vi "Demultiplexer_Laser160.vi"() -> ()   [LabVIEW 2012]
uses:
  <vilib>/Platform/TimedLoop/XDataNode/timing_clust.ctl
  <vilib>/Platform/TimedLoop/XDataNode/nitl_modes.ctl
  <vilib>/Platform/TimedLoop/XDataNode/wakeup.ctl
  <vilib>/rvi/Emulation/niFpgaSctlEmulationRegisterWithScheduler.vi
  <vilib>/rvi/eio/common/nirviEmuTemplateMethod_errors.vi
  <vilib>/rvi/Emulation/niFpgaSctlEmulationScheduler.vi
  <vilib>/rvi/FIFO/Fifo_Resource/nirvififoEmulationSetSize.vi
  <vilib>/rvi/DataTransferAndStorage/Container/Common/niFpgaContainerGetUniqueNameForEmu.vi
  <vilib>/rvi/errors/niFpgaSetErrorForExecOnDevCompSimple.vi
  <vilib>/rvi/eio/common/nirviEmuReportErrorAndStop.vi
  <vilib>/rvi/Emulation/niFpgaSctlEmulationFifoFullMgr.vi
  <vilib>/rvi/Emulation/niFpgaSctlEmulationResourceMgr.vi
  <vilib>/rvi/interface/RandomDataEmulation/nirviRandomDataFPGAFIFO.vi
  <vilib>/rvi/interface/RandomDataEmulation/niFpgaRandomDataHandleErrors.vi
  <vilib>/rvi/Emulation/niFpgaSctlEmulationGlobalWrite.vi
  <vilib>/Platform/TimedLoop/XDataNode/XDataNode.xnode
  <vilib>/eio/EIONode/EIONode.xnode
  <vilib>/rvi/DataTransferAndStorage/Container/XNode/niFpgaContainer.xnode
  <vilib>/rvi/FIFO/Fifo_Resource/nirvififoEmulationClear.vi
  <vilib>/rvi/FIFO/Fifo_Resource/nirvififoEmulationWrite.vi
  <vilib>/rvi/FIFO/Fifo_Resource/nirvififoEmulationRead.vi
  <vilib>/rvi/interface/RandomDataEmulation/nirviRandomDataFpgaReadWriteTemplate.vi
  <vilib>/Platform/TimedLoop/XDataNode/XDNodeRunTimeDep.lvlib
panel:
  out "Laser pulse count A1":u16
  out "ToHost FIFO Overflow A2Ch2":bool
  out "ToHost FIFO Overflow A2Ch1":bool
  out "ToHost FIFO Overflow A1Ch2":bool
  in  "Samples per pixel Acq A2":u16=10000 caption="Samples per pixel Acq"
  in  "Samples per pixel Acq A1":u16=10000 caption="Samples per pixel Acq"
  in  "Requested pixels A2":u32=100000 caption="Requested pixels"
  in  "Samples per pixel A2":u16=10000 caption="Samples per pixel"
  out "ToHost FIFO Overflow A1Ch1":bool
  out "Acquiring":bool
  in  "Wait for trigger":bool
  in  "Acquire continuously":bool=TRUE
  in  "Requested pixels A1":u32=100000 caption="Requested pixels"
  in  "Clear Interloop FIFO":bool
  out "Interloop FIFO overflow":bool
  in  "Samples per pixel A1":u16=10000 caption="Samples per pixel"
  in  "Acquire":bool
  out "Interloop FIFO timeout":bool
  in  "Commit":bool
  out "Xpoint_Switch_Ready":bool
  in  "Xpoint_Switch_Write":bool
  in  "Clock Source":u8(ring)=3 items=["Tristate"=0, "Sync Clock (PXIe only)"=2, "Adapter Module Onboard Clock"=3, "Strobe from Crosspoint Switch"=4, "Strobe Bypass"=5]
  in  "Onboard_Clock_Write":bool
  in  "Onboard_Clock_Write_Data":u16
  out "Onboard_Clock_Ready":bool
  in  "Acq_Reset":bool
  # "6587 IO module configuration"
  # "Demultiplexer - Laser 160MHz"
  # "Acquisition control"
  # "Area 1"
  # "Area 2"
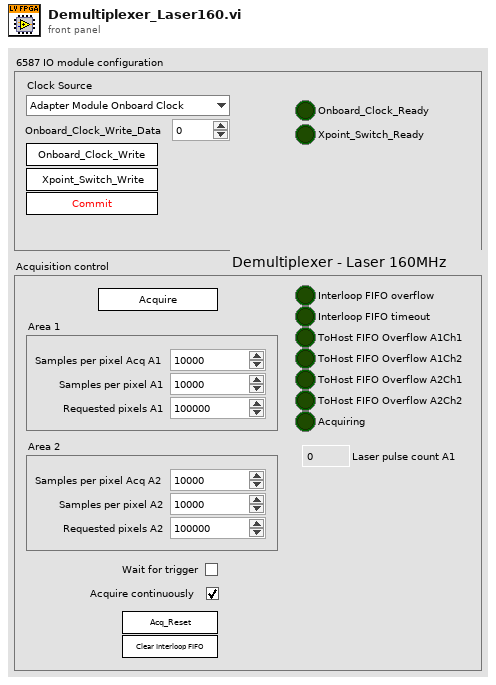
[diagram p1: front panel]
types:
  T1 = typedef "XDNodeRunTimeDep.lvlib/timing_clust.ctl" = cluster{"Expected End [f-1]":u64, "Actual End [f-1]":u64, "Finished Late? [f-1]":bool, "Expected End [i-1]":u64, "Actual End [i-1]":u64, "Finished Late? [i-1]":bool, "Expected Start [i]":u64, "Actual Start [i]":u64, "Expected Start [f]":u64, "Actual Start [f]":u64, "Source Name":string, "Structure Name":string, "Period":i64, "Deadline":i64, "Offset":i64, "Start":i64, "Priority":i32, "Timeout":i32, "Mode":T2, "Wakeup Reason":T3, "Error":errorcluster, "Source Type":string, "Secondary Source Type":string, "Global End Time":u64, "Global Start Time":u64, "Frame Duration":u64, "Iteration Duration":u64, "Assigned CPU":i32, "I/O Scan Engine Mode":u32}
  T2 = typedef "XDNodeRunTimeDep.lvlib/nitl_modes.ctl" = enum32{"No Change", "Process missed periods, maintain original phase", "Discard missed periods, maintain original phase", "Process missed periods, ignore original phase", "Discard missed periods, ignore original phase"}
  T3 = typedef "XDNodeRunTimeDep.lvlib/wakeup.ctl" = enum32{"Normal", "Aborted", "Asynchronous wakeup", "Timing source error", "Timed loop error", "Timeout"}
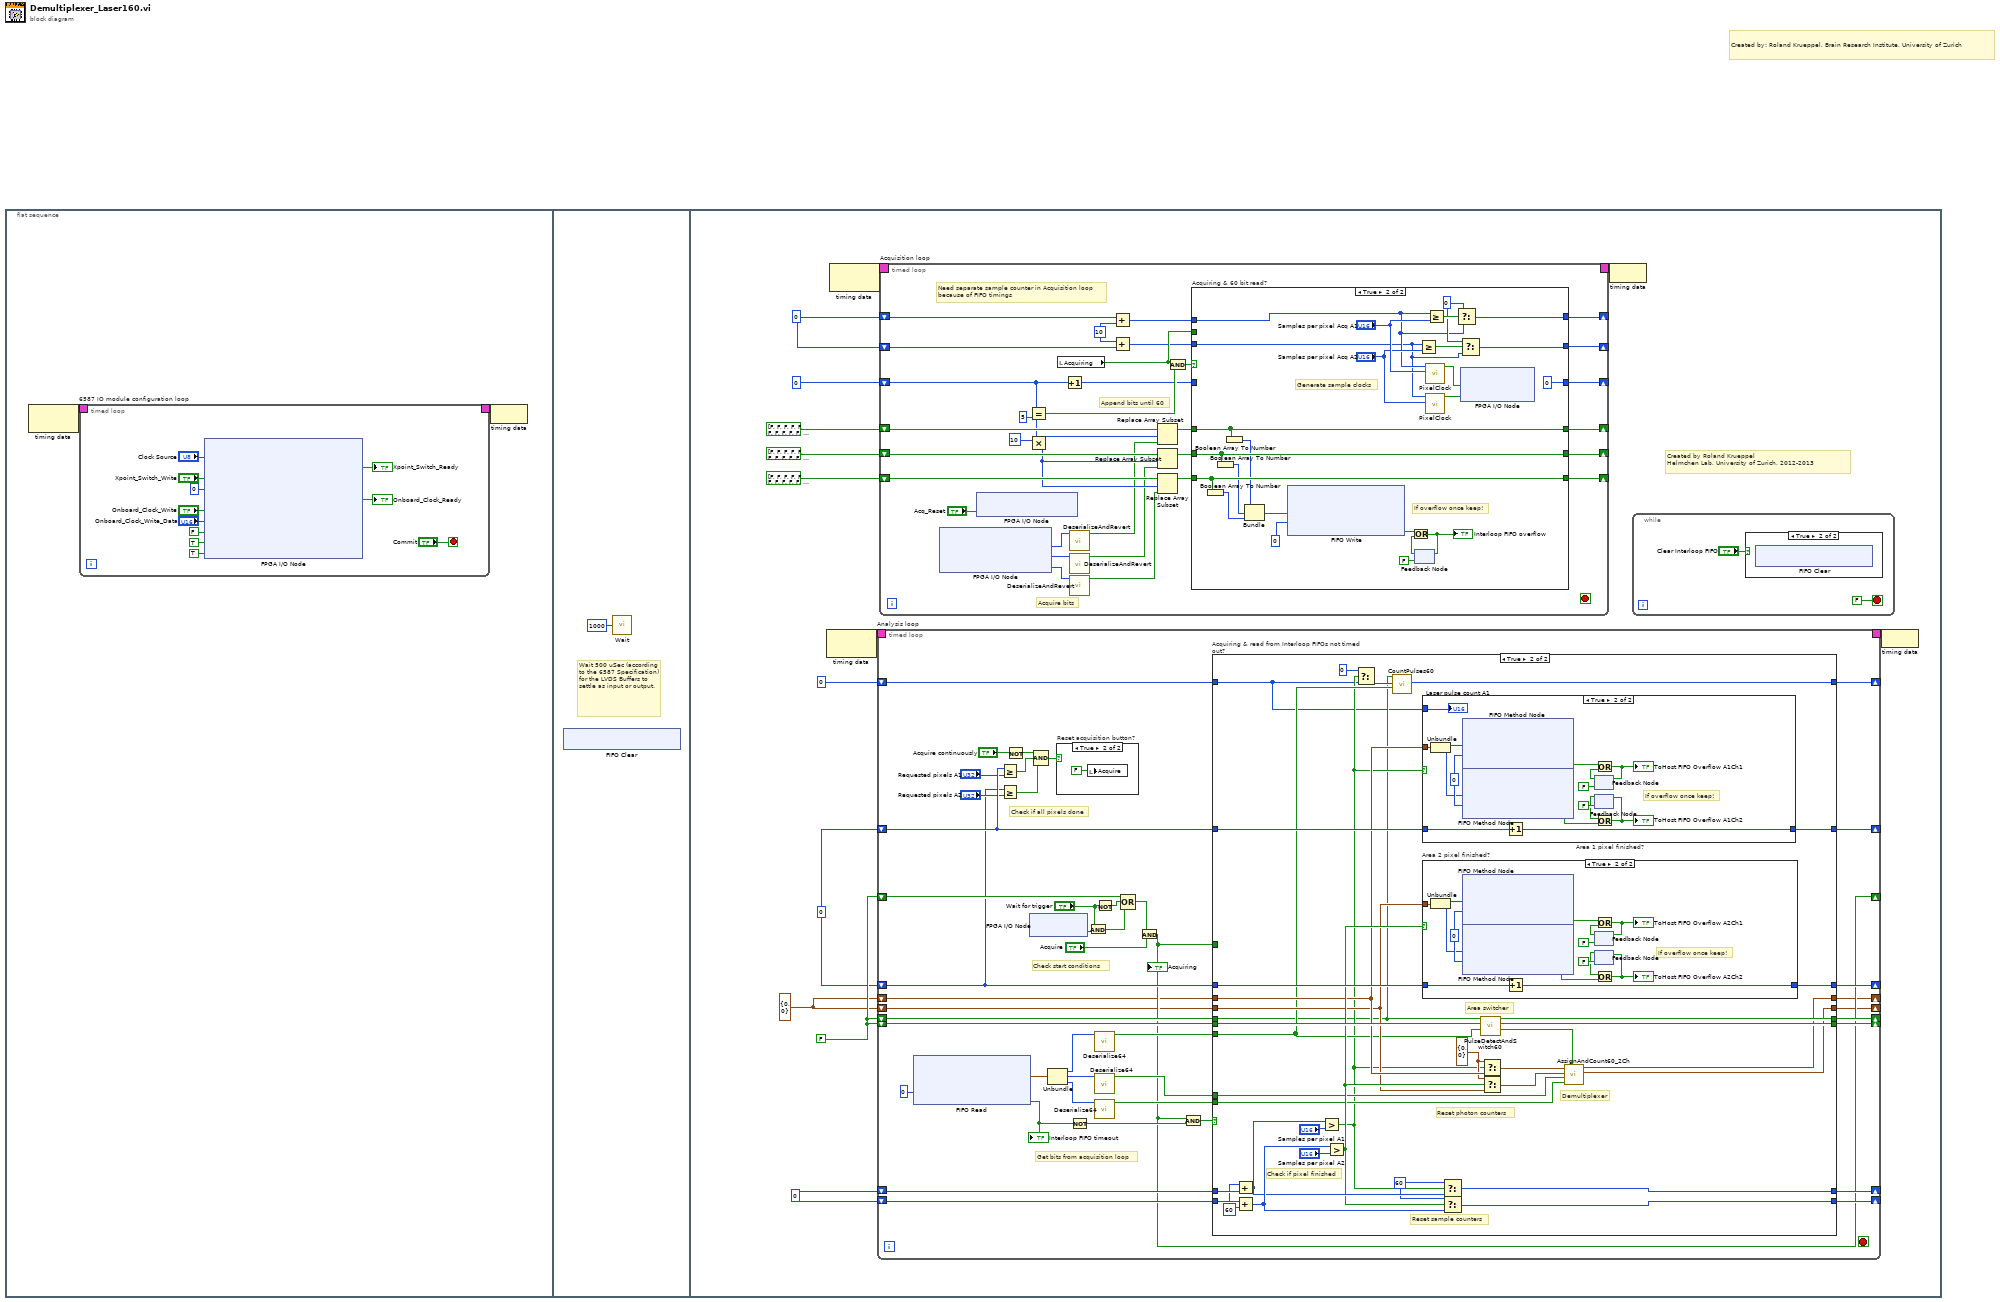
[diagram p0: block diagram]
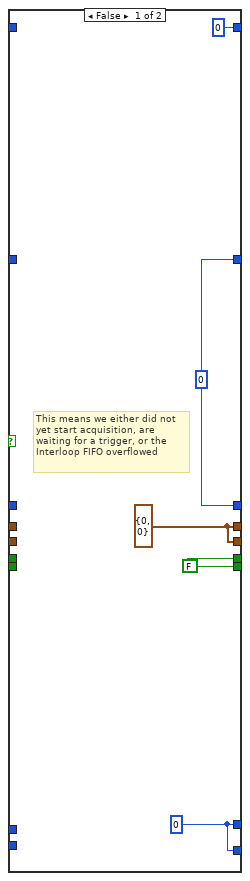
[diagram p5: hidden frame]
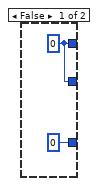
[diagram p9: hidden frame]
diagram:
  # "Created by: Roland Krueppel, Brain Research Institute, University of Zurich"
  n1 = flat-sequence {
    frame #0 {
      n2 = node-c288() -> (w2:T1)  [unwired: 1 in]
      n3 = timed-loop "6587 IO module configuration loop" {
        timing: w2 -> [_]
        timing-out: [_] -> w1
        stop <- "Commit" stop-if-true
        n4 = xnode "FPGA I/O Node"("IO Module\\Acq_IO_Clock_Source"="Clock Source", "IO Module\\Xpoint_Switch_Write"="Xpoint_Switch_Write", "IO Module\\LVDS_Data_Dir"=u16 0 ("IO Module\\LVDS_Data_Dir"), "IO Module\\Onboard_Clock_Write"="Onboard_Clock_Write", "IO Module\\Onboard_Clock_Write_Data"="Onboard_Clock_Write_Data", "IO Module\\SE_PFI0_WE"=FALSE ("IO Module\\SE_PFI0_WE"), "IO Module\\SE_PFI1_WE"=TRUE ("IO Module\\SE_PFI1_WE"), "IO Module\\SE_PFI2_WE"=TRUE ("IO Module\\SE_PFI2_WE")) -> ("IO Module\\Xpoint_Switch_Ready"=→"Xpoint_Switch_Ready":bool, "IO Module\\Onboard_Clock_Ready"=→"Onboard_Clock_Ready":bool)  [unwired: 10 in, 10 out]
      }
      n5 = node-c288(w1) -> ()
    }
    frame #1 {
      # "Wait 500 uSec (according to the 6587 Specification) for the LVDS Buffers to settle as input or output."
      n6 = xnode "FIFO Clear"() -> ()  [unwired: 1 in, 1 out]
      n7 = call "Wait"("Count(uSec)"=u32 1000) -> ()  [unwired: 1 out]
    }
    frame #2 {
      w21 = cluster{u16, u16} {0, 0} ("output cluster")
      w22 = u16 0
      w20 = u32 0 ("Cycle counter out")
      w23 = u16 0
      w24 = FALSE ("Last laser bit out")
      # "Created by Roland Krueppel\nHelmchen Lab, University of Zurich, 2012-2013"
      n8 = node-c288() -> (w30:T1)  [unwired: 1 in]
      n9 = node-c288() -> (w32:T1)  [unwired: 1 in]
      n10 = timed-loop "Analysis loop" {
        timing: w30 -> [_]
        timing-out: [_] -> w29
        shift-right: [w75] -> _
        shift-left: w24 -> [w78]
        shift-right: [w77] -> _
        shift-left: w24 -> [w76]
        shift-right: [w51] -> _
        shift-left: w23 -> [w74]
        shift-right: [w49] -> _
        shift-left: w20 -> [w73]
        shift-right: [w47] -> _
        shift-left: w24 -> [w62]
        shift-right: [w50] -> _
        shift-left: w23 -> [w57]
        shift-right: [w48] -> _
        shift-left: w20 -> [w55]
        shift-right: [w38] -> _
        shift-left: w21 -> [w40]
        shift-right: [w37] -> _
        shift-left: w21 -> [w39]
        shift-right: [w36] -> _
        shift-left: u16 0 ("New pulse count") -> [w35]
        stop <- _ stop-if-true
        # "Get bits from acquisition loop"
        # "Check start conditions"
        # "Check if all pixels done"
        n11 = xnode ("FIFO Read")("Timeout"=0) -> ("Element"=w44:cluster{"Laser":u64, "Ch0":u64, "Ch1":u64}, "Timed Out?"=w45:bool)  [unwired: 1 in, 1 out]
        "Interloop FIFO timeout" <- w45
        n12 = Greater Or Equal?(x=w73, y="Requested pixels A1") -> (x >= y?=w53:bool)
        n13 = Greater Or Equal?(x=w55, y="Requested pixels A2") -> (x >= y?=w52:bool)
        n14 = Not(x="Acquire continuously") -> (.not. x?=w54:bool)
        n15 = xnode "FPGA I/O Node"() -> ("TriggerIn"=w68:bool)  [unwired: 1 in, 1 out]
        n16 = Compound Arithmetic op=AND(w54, w53, w52) -> (w70:bool)
        n17 = Unbundle(w44) -> ("Laser"=w43:u64, "Ch0"=w42:u64, "Ch1"=w41:u64)
        n18 = case "Reset acquisition button?" shown="True" w70 {
          frame False {
          }
          frame True {
            n19 = local write "Acquire"(FALSE ("Acquire")) -> ()
          }
        }
        n20 = Not(x=w45) -> (.not. x?=w63:bool)
        n21 = And(x="Wait for trigger", y=w68) -> (x .and. y?=w65:bool)
        n22 = call "Deserialize64.vi"("U64 input"=w43) -> ("60bit output"=w60:bool[])  [unwired: 10 in]
        n23 = call "Deserialize64.vi"("U64 input"=w42) -> ("60bit output"=w59:bool[])  [unwired: 10 in]
        n24 = call "Deserialize64.vi"("U64 input"=w41) -> ("60bit output"=w58:bool[])  [unwired: 10 in]
        n25 = Not(x="Wait for trigger") -> (.not. x?=w66:bool)
        n26 = Compound Arithmetic op=OR(w62, w66, w65) -> (w64:bool)
        n27 = And(x=w64, y="Acquire") -> (x .and. y?=w47:bool)
        "Acquiring" <- w47
        n28 = And(x=w47, y=w63) -> (x .and. y?=w61:bool)
        n29 = case "Acquiring & read from Interloop FIFOs not timed out?" shown="True" w61 {
          tunnel: w78 -> [w93 w133]
          tunnel: w40 -> [w97 w129]
          tunnel: [w92 w132] -> w77
          tunnel: w76 -> [w94 w114]
          tunnel: [w91 w131] -> w75
          tunnel: w74 -> [w96 w147]
          tunnel: w73 -> [w95 w143]
          tunnel: w60 -> [_ w119]
          tunnel: w59 -> [_ w124]
          tunnel: w47 -> [w98 _]
          tunnel: w58 -> [_ w123]
          tunnel: w57 -> [w85 w145]
          tunnel: w55 -> [w88 w142]
          tunnel: [w86 w135] -> w51
          tunnel: [w84 w137] -> w50
          tunnel: [w90 w121] -> w38
          tunnel: [w89 w140] -> w49
          tunnel: [w87 w141] -> w48
          tunnel: w39 -> [w83 w126]
          tunnel: [w82 w120] -> w37
          tunnel: [w80 w118] -> w36
          tunnel: w35 -> [w81 w113]
          frame False {
            n30 = case "Acquiring?" shown="True" w98 {
              tunnel: w97 -> [_ w110]
              tunnel: w96 -> [_ w107]
              tunnel: w95 -> [_ w109]
              tunnel: w94 -> [_ w112]
              tunnel: w93 -> [_ w111]
              tunnel: [w103 w112] -> w92
              tunnel: [w103 w111] -> w91
              tunnel: [w101 w110] -> w90
              tunnel: [w102 w109] -> w89
              tunnel: w88 -> [_ w108]
              tunnel: [w102 w108] -> w87
              tunnel: [w100 w107] -> w86
              tunnel: [w100 w106] -> w84
              tunnel: w85 -> [_ w106]
              tunnel: w83 -> [_ w105]
              tunnel: [w101 w105] -> w82
              tunnel: w81 -> [_ w104]
              tunnel: [u16 0 ("New pulse count") w104] -> w80
              frame False {
                w101 = cluster{u16, u16} {0, 0} ("output cluster")
                w102 = u32 0 ("Cycle counter out")
                w100 = u16 0
                w103 = FALSE ("Last laser bit out")
                # "This means we either did not\nyet start acquisition, are\nwaiting for a trigger, or the\nInterloop FIFO overflowed"
              }
              frame True {
                # "This means we are\nreading faster here\nthan acquiring in\nAcquisition loop\n-> keep all values"
              }
            }
          }
          frame True {
            w122 = cluster{u16, u16} {0, 0} ("t")
            w134 = u16 60 ("t")
            w144 = u16 60
            # "Demultiplexer"
            # "Reset photon counters"
            # "Area switcher"
            # "Check if pixel finished"
            # "Reset sample counters"
            n31 = Add(x=w144, y=w147) -> (x+y=w136:u16)
            n32 = Add(x=w145, y=w144) -> (x+y=w138:u16)
            n33 = Greater?(x=w136, y="Samples per pixel A1") -> (0:w117:bool)
            n34 = Greater?(x=w138, y="Samples per pixel A2") -> (0:w130:bool)
            n35 = Select(t=u16 0, s=w117, f=w113) -> (s? t:f=w116:u16)
            n36 = call "CountPulses60.vi"("60bit input"=w119, "Previous pulse count"=w116, "Last sample"=w114) -> ("New pulse count"=w118:u16)  [unwired: 7 in, 1 out]
            n37 = case "Area 1 pixel finished?" shown="True" w117 {
              tunnel: w129 -> [_ w175]
              tunnel: w143 -> [w163 w177]
              tunnel: [w163 w176] -> w140
              tunnel: w113 -> [_ w172]
              frame False {
              }
              frame True {
                w178 = 0 ("Timeout")
                # "If overflow once keep!"
                n38 = Unbundle(w175) -> (w174:u16, w173:u16)
                n39 = xnode ("FIFO Method Node")("Element"=w174, "Timeout"=w178) -> ("Timed Out?"=w167:bool)  [unwired: 1 in, 1 out]
                n40 = xnode ("FIFO Method Node")("Element"=w173, "Timeout"=w178) -> ("Timed Out?"=w166:bool)  [unwired: 1 in, 1 out]
                n41 = Increment(x=w177) -> (x+1=w176:u32)
                n42 = feedback #1(FALSE) -> (w171:bool)
                n43 = feedback #2(FALSE) -> (w168:bool)
                n44 = Or(x=w167, y=w171) -> (x .or. y?=w165:bool)
                "ToHost FIFO Overflow A1Ch1" <- w165
                n45 = feedback-in #1(w165) -> ()
                n46 = Or(x=w168, y=w166) -> (x .or. y?=w164:bool)
                "ToHost FIFO Overflow A1Ch2" <- w164
                n47 = feedback-in #2(w164) -> ()
                "Laser pulse count A1" <- w172
              }
            }
            n48 = case "Area 2 pixel finished?" shown="True" w130 {
              tunnel: w142 -> [w148 w161]
              tunnel: [w148 w160] -> w141
              tunnel: w126 -> [_ w159]
              frame False {
              }
              frame True {
                w162 = 0 ("Timeout")
                # "If overflow once keep!"
                n49 = Unbundle(w159) -> (w158:u16, w157:u16)
                n50 = xnode ("FIFO Method Node")("Element"=w158, "Timeout"=w162) -> ("Timed Out?"=w152:bool)  [unwired: 1 in, 1 out]
                n51 = xnode ("FIFO Method Node")("Element"=w157, "Timeout"=w162) -> ("Timed Out?"=w151:bool)  [unwired: 1 in, 1 out]
                n52 = Increment(x=w161) -> (x+1=w160:u32)
                n53 = feedback #3(FALSE) -> (w156:bool)
                n54 = feedback #4(FALSE) -> (w153:bool)
                n55 = Or(x=w152, y=w156) -> (x .or. y?=w150:bool)
                "ToHost FIFO Overflow A2Ch1" <- w150
                n56 = feedback-in #3(w150) -> ()
                n57 = Or(x=w153, y=w151) -> (x .or. y?=w149:bool)
                "ToHost FIFO Overflow A2Ch2" <- w149
                n58 = feedback-in #4(w149) -> ()
              }
            }
            n59 = Select(t=w134, s=w117, f=w136) -> (s? t:f=w135:u16)
            n60 = Select(t=w134, s=w130, f=w138) -> (s? t:f=w137:u16)
            n61 = call "PulseDetectAndSwitch60.vi"("Laser bits in"=w119, "Last area"=w133, "Last laser bit in"=w114) -> ("Area bits out"=w128:bool[], "New last area out"=w131:bool, "New last laser bit out"=w132:bool)  [unwired: 6 in]
            n62 = Select(t=w122, s=w117, f=w129) -> (s? t:f=w127:cluster{u16, u16})
            n63 = Select(t=w122, s=w130, f=w126) -> (s? t:f=w125:cluster{u16, u16})
            n64 = call "AssignAndCount60_2Ch.vi"("Area bits in"=w128, "PMT bits Ch2 in"=w123, "PMT bits Ch1 in"=w124, "Photon counters area 2 in"=w125, "Photon counters area 1 in"=w127) -> ("Photon counters area 2 out"=w120:cluster{u16, u16}, "Photon counters area 1 out"=w121:cluster{u16, u16})  [unwired: 5 in]
          }
        }
      }
      n65 = timed-loop "Acquisition loop" {
        timing: w32 -> [_]
        timing-out: [_] -> w31
        shift-right: [w205] -> _
        shift-left: bool[] [FALSE, FALSE, FALSE, FALSE, FALSE, FALSE, FALSE, FALSE, FALSE, FALSE, FALSE, FALSE, FALSE, FALSE, FALSE, FALSE, FALSE, FALSE, FALSE, FALSE, FALSE, FALSE, FALSE, FALSE, FALSE, FALSE, FALSE, FALSE, FALSE, FALSE, FALSE, FALSE, FALSE, FALSE, FALSE, FALSE, FALSE, FALSE, FALSE, FALSE, FALSE, FALSE, FALSE, FALSE, FALSE, FALSE, FALSE, FALSE, FALSE, FALSE, FALSE, FALSE, FALSE, FALSE, FALSE, FALSE, FALSE, FALSE, FALSE, FALSE, FALSE, FALSE, FALSE, FALSE] ("Boolean array") -> [w213]
        shift-right: [w204] -> _
        shift-left: bool[] [FALSE, FALSE, FALSE, FALSE, FALSE, FALSE, FALSE, FALSE, FALSE, FALSE, FALSE, FALSE, FALSE, FALSE, FALSE, FALSE, FALSE, FALSE, FALSE, FALSE, FALSE, FALSE, FALSE, FALSE, FALSE, FALSE, FALSE, FALSE, FALSE, FALSE, FALSE, FALSE, FALSE, FALSE, FALSE, FALSE, FALSE, FALSE, FALSE, FALSE, FALSE, FALSE, FALSE, FALSE, FALSE, FALSE, FALSE, FALSE, FALSE, FALSE, FALSE, FALSE, FALSE, FALSE, FALSE, FALSE, FALSE, FALSE, FALSE, FALSE, FALSE, FALSE, FALSE, FALSE] ("Boolean array") -> [w212]
        shift-right: [w203] -> _
        shift-left: 0 -> [w202]
        shift-right: [w198] -> _
        shift-left: bool[] [FALSE, FALSE, FALSE, FALSE, FALSE, FALSE, FALSE, FALSE, FALSE, FALSE, FALSE, FALSE, FALSE, FALSE, FALSE, FALSE, FALSE, FALSE, FALSE, FALSE, FALSE, FALSE, FALSE, FALSE, FALSE, FALSE, FALSE, FALSE, FALSE, FALSE, FALSE, FALSE, FALSE, FALSE, FALSE, FALSE, FALSE, FALSE, FALSE, FALSE, FALSE, FALSE, FALSE, FALSE, FALSE, FALSE, FALSE, FALSE, FALSE, FALSE, FALSE, FALSE, FALSE, FALSE, FALSE, FALSE, FALSE, FALSE, FALSE, FALSE, FALSE, FALSE, FALSE, FALSE] ("Boolean array") -> [w201]
        shift-right: [w197] -> _
        shift-left: w22 -> [w187]
        shift-right: [w196] -> _
        shift-left: w22 -> [w185]
        stop <- _ stop-if-true
        w183 = u16 10 ("y")
        # "Need separate sample counter in Acquisition loop\nbecause of FIFO timings"
        # "Append bits until 60"
        # "Acquire bits"
        n66 = xnode "FPGA I/O Node"() -> ("IO Module\\LVDS_Ch0_Rd"=w193:u16, "IO Module\\LVDS_Ch1_Rd"=w191:u16, "IO Module\\LVDS_Ch2_Rd"=w189:u16)  [unwired: 3 in, 3 out]
        n67 = xnode "FPGA I/O Node"("IO Module\\Acq_Reset"="Acq_Reset") -> ()  [unwired: 1 in, 1 out]
        n68 = Equal?(x=w202, y=5) -> (x = y?=w209:bool)
        n69 = Multiply(x=10 ("y"), y=w202) -> (x*y=w200:i32)
        n70 = local read "Acquiring"() -> (w195:bool)
        n71 = Increment(x=w202) -> (x+1=w194:i32)
        n72 = call "DeserializeAndRevert.vi"("U16 input"=w193) -> ("10bit output"=w192:bool[])  [unwired: 10 in]
        n73 = call "DeserializeAndRevert.vi"("U16 input"=w191) -> ("10bit output"=w190:bool[])  [unwired: 10 in]
        n74 = call "DeserializeAndRevert.vi"("U16 input"=w189) -> ("10bit output"=w188:bool[])  [unwired: 10 in]
        n75 = Add(x=w187, y=w183) -> (x+y=w186:u16)
        n76 = Add(x=w183, y=w185) -> (x+y=w184:u16)
        n77 = Replace Array Subset(array=w213, new element=w192, index=w200) -> (w207:bool[])
        n78 = Replace Array Subset(array=w212, new element=w190, index=w200) -> (w206:bool[])
        n79 = Replace Array Subset(array=w201, new element=w188, index=w200) -> (w199:bool[])
        n80 = And(x=w195, y=w209) -> (x .and. y?=w208:bool)
        n81 = case "Acquiring & 60 bit read?" shown="True" w208 {
          tunnel: w207 -> [w224 w250]
          tunnel: w206 -> [w223 w252]
          tunnel: [w224 w250] -> w205
          tunnel: [w223 w252] -> w204
          tunnel: [w215 0] -> w203
          tunnel: w194 -> [w216 _]
          tunnel: w199 -> [w222 w251]
          tunnel: [w222 w251] -> w198
          tunnel: w186 -> [w220 w235]
          tunnel: [w217 w248] -> w197
          tunnel: w184 -> [w219 w234]
          tunnel: [w218 w243] -> w196
          tunnel: w195 -> [w221 _]
          frame False {
            n82 = case "Acquiring?" shown="True" w221 {
              tunnel: w220 -> [_ w229]
              tunnel: w219 -> [_ w228]
              tunnel: [w226 w229] -> w217
              tunnel: [w226 w228] -> w218
              tunnel: w216 -> [_ w227]
              tunnel: [0 w227] -> w215
              frame False {
                w226 = u16 0
              }
              frame True {
              }
            }
          }
          frame True {
            w244 = u16 0 ("t")
            # "If overflow once keep!"
            # "Generate sample clocks"
            n83 = Boolean Array To Number(Boolean array=w251) -> (number=w238:u64)
            n84 = Boolean Array To Number(Boolean array=w252) -> (number=w239:u64)
            n85 = Boolean Array To Number(Boolean array=w250) -> (number=w240:u64)
            n86 = Bundle(w240, w239, w238) -> (w237:cluster{u64, u64, u64})  [unwired: 1 in]
            n87 = xnode ("FIFO Write")("Element"=w237, "Timeout"=0) -> ("Timed Out?"=w233:bool)  [unwired: 1 in, 1 out]
            n88 = feedback #5(FALSE) -> (w231:bool)
            n89 = Or(x=w233, y=w231) -> (x .or. y?=w232:bool)
            "Interloop FIFO overflow" <- w232
            n90 = feedback-in #5(w232) -> ()
            n91 = Greater Or Equal?(x=w234, y="Samples per pixel Acq A2") -> (x >= y?=w245:bool)
            n92 = call "PixelClock.vi"("Samples per pixel"="Samples per pixel Acq A1", "Sample counter"=w235) -> ("Pixel clock"=w246:bool)  [unwired: 9 in]
            n93 = call "PixelClock.vi"("Samples per pixel"="Samples per pixel Acq A2", "Sample counter"=w234) -> ("Pixel clock"=w241:bool)  [unwired: 9 in]
            n94 = Greater Or Equal?(x=w235, y="Samples per pixel Acq A1") -> (x >= y?=w249:bool)
            n95 = Select(t=w244, s=w249, f=w235) -> (s? t:f=w248:u16)
            n96 = Select(t=w244, s=w245, f=w234) -> (s? t:f=w243:u16)
            n97 = xnode "FPGA I/O Node"("Pixel clock A1"=w246, "Pixel clock A2"=w241) -> ()  [unwired: 2 in, 2 out]
          }
        }
      }
      n98 = node-c288(w31) -> ()
      n99 = while {
        stop <- FALSE stop-if-true
        n100 = case shown="True" "Clear Interloop FIFO" {
          frame False {
          }
          frame True {
            n101 = xnode ("FIFO Clear")() -> ()  [unwired: 1 in, 1 out]
          }
        }
      }
      n102 = node-c288(w29) -> ()
    }
  }
